vi "Initialize.vi"(5 "Buffer Capacity":i32=102400, 7 "Maximum Messages":i32=-1, 8 "Error In":errorcluster) -> (0 "Error Out":errorcluster)   [LabVIEW 2017, in "Toolkit.lvlib"]
doc: "Initializes all internal buffers and the default log file."
uses:
  Toolkit.lvlib
  Support/Action.ctl
  Support/File/File Action.ctl
  Support/Control Action.ctl
  Support/Error/Error Action.ctl
  Support/File/File.lvlib
  Support/Error/Error.lvlib
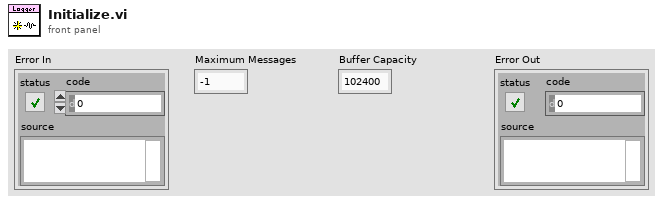
[diagram p1: front panel]
types:
  T1 = typedef "Toolkit.lvlib/Error.lvlib/Error Action.ctl" = enum16{"Initialize", "Get", "Set Verbosity", "Set User-Defined Codes", "Set User-Defined Descriptions", "Shutdown"}
  T2 = typedef "Toolkit.lvlib/Control Action.ctl" = enum16{"Initialize", "Get", "Set", "Shutdown"}
  T3 = typedef "Toolkit.lvlib/File.lvlib/File Action.ctl" = enum16{"Initialize", "Set Maximum File Size", "Set Maximum File Count", "Set Root Folder", "Set Enable Calendar Folder Tree", "Set File Extension", "Start", "Write", "Stop", "Shutdown"}
  T4 = typedef "Toolkit.lvlib/Action.ctl" = enum16{"Initialize", "Register", "Log", "Unregister", "Set Level", "Shutdown"}
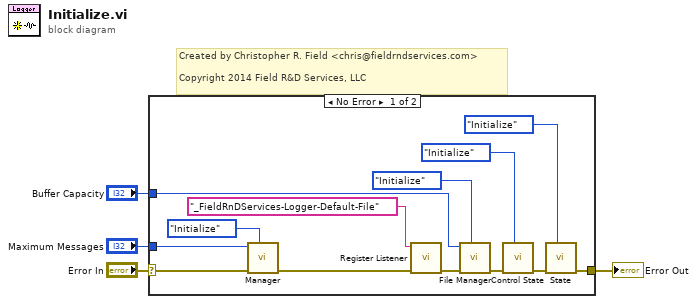
[diagram p0: block diagram]
diagram:
  # "Created by Christopher R. Field <chris@fieldrndservices.com>\n\nCopyright 2014 Field R&D Services, LLC"
  n1 = case shown="No Error" "Error In" {
    selector: "Error In" -> [w16 w18]
    tunnel: [w8 w18] -> w3
    tunnel: "Maximum Messages" -> [w6 _]
    tunnel: "Buffer Capacity" -> [w5 _]
    frame No Error {
      n2 = call "Manager.vi"("Action"=Action."Initialize", "Error In"=w16, "Value In"=w6) -> ("Error Out"=w15:errorcluster)  [unwired: 8 in]
      n3 = call "Register Listener.vi"("Error In"=w15, "Listener ID"="_FieldRnDServices-Logger-Default-File") -> ("Error Out"=w9:errorcluster)  [unwired: 9 in]
      n4 = call "File Manager.vi"("Action"=File_Action."Initialize", "Error In"=w9, "Set Value"=w5) -> ("Error Out"=w13:errorcluster)  [unwired: 8 in]
      n5 = call "Control State.vi"("Action"=Control_Action."Initialize", "Error In"=w13) -> ("Error Out"=w11:errorcluster)  [unwired: 8 in, 1 out]
      n6 = call "State.vi"("Action"=Error_Action."Initialize", "Error In"=w11) -> ("Error Out"=w8:errorcluster)  [unwired: 8 in, 1 out]
    }
    frame Error {
    }
  }
  "Error Out" <- w3
